vi "Boiler Controller.vi"(8 "error in (no error)":errorcluster, 11 "Message Queues":T1) -> (0 "error out":errorcluster)   [LabVIEW 2015]
uses:
  support/Message Queue/All Message Queues.ctl
  support/Message Queue/Message Cluster.ctl
  support/Message Queue/Message Queue.lvlib
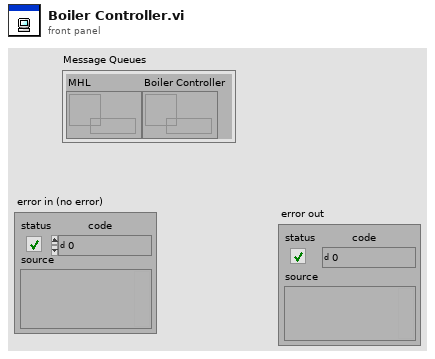
[diagram p1: front panel]
types:
  T1 = typedef "Message Queue.lvlib/All Message Queues.ctl" = cluster{"MHL":refnum<queue>, "Boiler Controller":refnum<queue>}
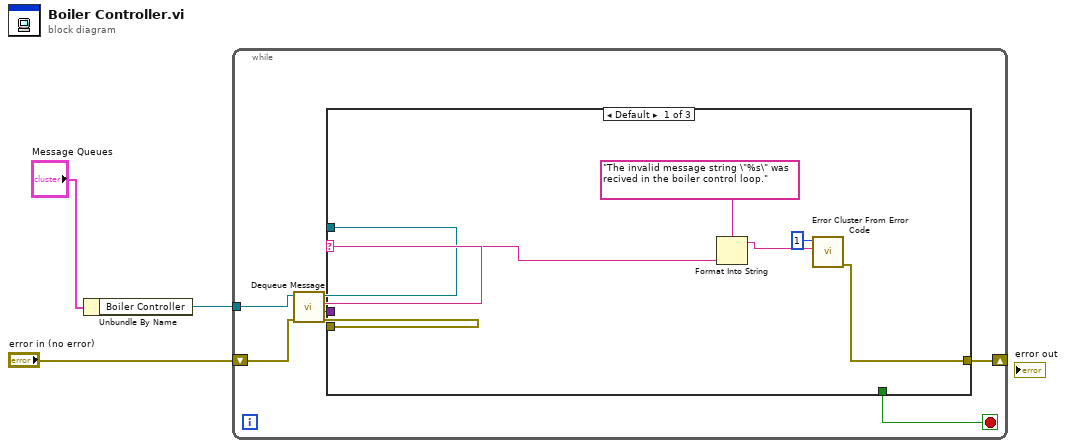
[diagram p0: block diagram]
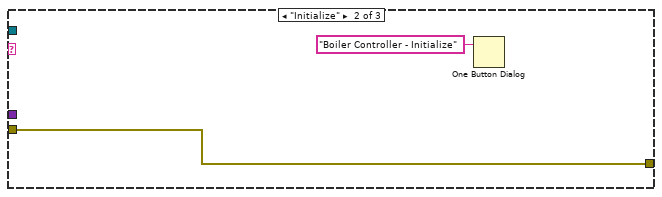
[diagram p2: hidden frame]
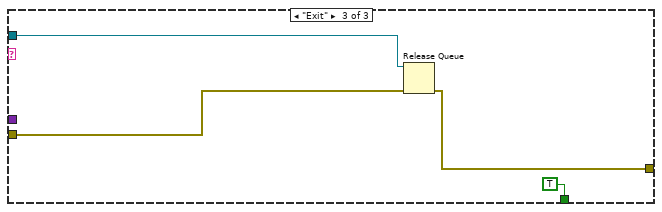
[diagram p3: hidden frame]
diagram:
  n1 = Unbundle By Name("Message Queues") -> ("Boiler Controller"=w2:refnum<queue>)
  n2 = while {
    tunnel: w2 -> [w11]
    shift-right: [w5] -> _
    shift-left: "error in (no error)" -> [w10]
    stop <- w4 stop-if-true
    n3 = call "Dequeue Message.vi"("error in (no error)"=w10, "Message Queue"=w11) -> ("error out"=w6:errorcluster, "Message Data"=w7:variant, "Message"=w9:string, "dup Message Queue"=w8:refnum<queue>)  [unwired: 6 in]
    n4 = case shown="Default" w9 {
      selector: w9 -> [w16 _ _]
      tunnel: w8 -> [_ _ w21]
      tunnel: w7 -> [_ _ _]
      tunnel: w6 -> [_ w17 w22]
      tunnel: [w12 w17 w20] -> w5
      tunnel: [_ _ TRUE] -> w4
      frame Default {
        n5 = Format Into String(format string="The invalid message string \"%s\" was recived in the boiler control loop.", w16) -> (resulting string=w14:string)  [unwired: 2 in, 1 out]
        n6 = call <vilib>:"Error Cluster From Error Code.vi"("error message (\"\")"=w14, "error code (0)"=1) -> ("error out"=w12:errorcluster)  [unwired: 7 in]
      }
      frame "Initialize" {
        n7 = One Button Dialog(message="Boiler Controller - Initialize") -> ()  [unwired: 1 in, 1 out]
      }
      frame "Exit" {
        n8 = Release Queue(queue=w21, error in (no error)=w22) -> (error out=w20:errorcluster)  [unwired: 1 in, 2 out]
      }
    }
  }
